vi "Main.vi"(8 "error in (no error)":errorcluster, 11 "ModuleAdmin":refnum<class "ModuleAdmin.lvclass">) -> ()   [LabVIEW 2018, in "FgenModule.lvlib"]
uses:
  FgenModule.lvlib
  <userlib>/NIST/ModuleAdminLib/ModuleAdmin/ModuleAdmin.lvclass
  C:/Program Files (x86)/National Instruments/LabVIEW 2018/user.lib/NIST/ModuleAdminLib/ModuleAdminBase/ModuleAdminBase.lvclass
  PublicAPI/Arguments/Requests/clStopArgument.ctl
  FgenPlugins/FgenPluginBaseClass/FgenPluginsBase.lvclass
  C:/Program Files (x86)/National Instruments/LabVIEW 2018/user.lib/NIST/BaseClasses/BasePlugin_class/BasePlugin.lvclass
  <userlib>/NIST/ModuleAdminLib/ModuleAdmin/ModuleAdmin.lvclass/ModuleAdmin.ctl
  FgenPlugins/FgenPluginBaseClass/FgenPluginsBase.lvclass/FgenPluginsBase.ctl
  MemberClasses/FunctionBaseClass/FunctionBase.lvclass/FunctionBase.ctl
  FgenPlugins/TypeDefs/clTriggers.ctl
  FgenPlugins/TypeDefs/Trigger.ctl
  FgenPlugins/TypeDefs/TriggerType.ctl
  <userlib>/NIST/BaseClasses/BasePlugin_class/BasePlugin.lvclass/BasePlugin.ctl
  FgenPlugins/TypeDefs/InitOptions.ctl
  FgenPlugins/TypeDefs/Channels.ctl
  FgenPlugins/TypeDefs/Channel.ctl
  <vilib>/Utility/error.llb/DialogType.ctl
  <userlib>/NIST/ModuleAdminLib/ModuleAdmin/Accessors/Read ShowPanel_.vi
  <userlib>/NIST/ModuleAdminLib/ModuleAdmin/Accessors/Write ShowPanel_.vi
  FgenPlugins/FgenPluginBaseClass/Accessors/Read FunctionClass.vi
  FgenPlugins/FgenPluginBaseClass/Accessors/Write FunctionClass.vi
  MemberClasses/FunctionBaseClass/Accessors/Write Waveforms.vi
  MemberClasses/FunctionBaseClass/Accessors/Read Waveforms.vi
  FgenPlugins/FgenPluginBaseClass/Accessors/Write Triggers.vi
  FgenPlugins/FgenPluginBaseClass/Read Triggers.vi
  <userlib>/NIST/BaseClasses/BasePlugin_class/Accessors/Read PluginIniFilePath.vi
  <userlib>/NIST/ModuleAdminLib/ModuleAdmin/Accessors/Read CloneRegRef.vi
  <extravilib>/ChannelInstances/Tag-bool/Read With Abort.vi
  <extravilib>/ChannelInstances/Tag-bool/Write With Abort.vi
  <extravilib>/ChannelInstances/Tag-bool/Instantiate.vi
  <extravilib>/ChannelInstances/Tag-bool/EndpointRead.vi
  <vilib>/Utility/error.llb/Error Cluster From Error Code.vi
  <extravilib>/ChannelInstances/Tag-bool/Endpoint.vi
  <vilib>/ErrorRing/Error Ring.xnode
  MemberClasses/FunctionBaseClass/FunctionBase.lvclass
  <userlib>/NIST/ModuleAdminLib/CloneRegistration/CloneRegistration.lvclass
  <userlib>/NIST/BaseClasses/Object_class/BaseObject.lvclass
  <userlib>/NIST/ModuleAdminLib/ModuleAdmin.lvlib
  FgenPlugins/FgenPlugins.lvlib
  <extravilib>/ChannelInstances/Tag-bool.lvlib
panel:
  out "error out":errorcluster
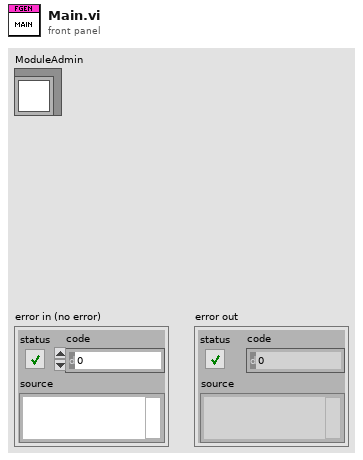
[diagram p1: front panel]
types:
  T1 = typedef "FgenModule.lvlib/clRequestEvents.ctl" = cluster{"StopRequest":refnum<user-event>, "PathToINI":refnum<user-event>, " LoadPlugin":refnum<user-event>, "ShowPanel":refnum<user-event>, "Initialize":refnum<user-event>, "GetChannels":refnum<user-event>, "SetChannels":refnum<user-event>, "Abort":refnum<user-event>, "Initiate":refnum<user-event>, "ConfigDlg":refnum<user-event>, "GetFunction":refnum<user-event>, "SetFunction":refnum<user-event>, "ConfigFunction":refnum<user-event>, "GetWfrm":refnum<user-event>, "SetWfrm":refnum<user-event>, "GetTriggers":refnum<user-event>, "SetTriggers":refnum<user-event>, "ConfigTriggers":refnum<user-event>, "Close":refnum<user-event>, "GetFunctionParams":refnum<user-event>, "SetFunctionParams":refnum<user-event>, "GetFunctionArbs":refnum<user-event>, "SetFunctionArbs":refnum<user-event>, "GetFunctionSampleRate":refnum<user-event>, "SetFunctionSampleRate":refnum<user-event>}
  T2 = typedef "FgenModule.lvlib/clBroadcastEvents.ctl" = cluster{"DidInit":refnum<user-event>, "StatusUpdate":refnum<user-event>, "ErrorReport":refnum<user-event>, "DidStop":refnum<user-event>, "PathToINI":refnum<user-event>, "Channels":refnum<user-event>, "Function":refnum<user-event>, "Waveforms":refnum<user-event>, "Triggers":refnum<user-event>, "FunctionParams":refnum<user-event>, "FunctionArbs":refnum<user-event>, "FunctionSampleRate":refnum<user-event>}
  T3 = typedef "FgenModule.lvlib/clStopArgument.ctl" = cluster{"Exit via Stop Module Req?":bool, "Wait for Module to stop?":bool, "ModuleAdmin":refnum<class "ModuleAdmin.lvclass">}
  T4 = enum32{"Invalid", "Standard", "Closed", "Hidden", "Minimized", "Maximized"}
  T5 = typedef "FgenPlugins.lvlib/clTriggers.ctl" = cluster{"Count":i32, "Triggers":T6[]}
  T6 = typedef "FgenPlugins.lvlib/Trigger.ctl" = cluster{"Source":string, "Slope":enum16{"Positive", "Negative", "Either"}, "Threshold":dbl, "Delay":dbl, "TriggerType":T7}
  T7 = typedef "FgenPlugins.lvlib/TriggerType.ctl" = enum16{"None", "Start", "Stop", "Hold", "Resume", "Advance"}
  T8 = typedef "FgenPlugins.lvlib/InitOptions.ctl" = cluster{"IDQuery":bool, "Reset":bool}
  T9 = typedef "FgenPlugins.lvlib/Channels.ctl" = cluster{"Count":u16, "Channel":T10[]}
  T10 = typedef "FgenPlugins.lvlib/Channel.ctl" = cluster{"Name":string, "Enabled":bool, "Operation":enum16{"Continuous", "Burst"}, "Impedance (50)":dbl, "Handle":string, "Connected":bool, "Mode (Function)":enum16{"Function", "Arbitrary", "Sequence"}}
  T11 = typedef "Tag-bool.lvlib/))Channel.ctl" = refnum<queue>
  T12 = typedef "DialogType.ctl" = u16
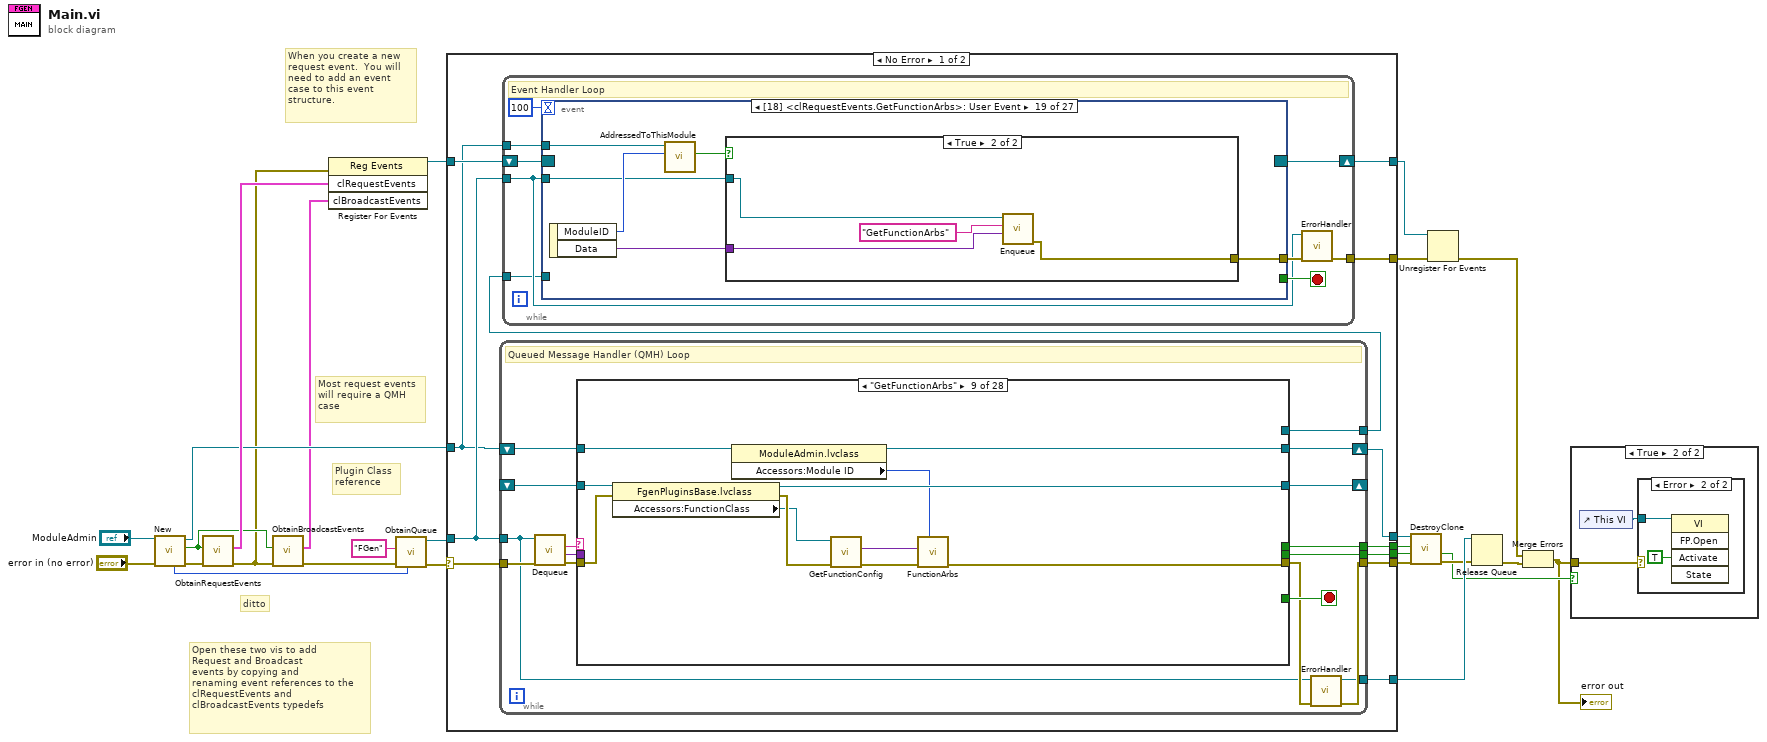
[diagram p0: block diagram]
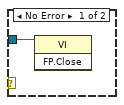
[diagram p3: hidden frame]
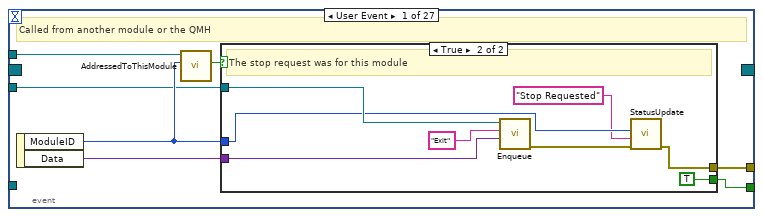
[diagram p4: hidden frame]
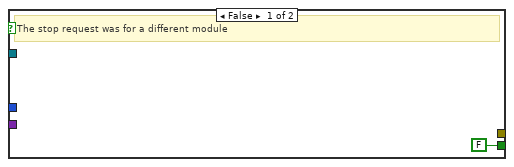
[diagram p5: hidden frame]
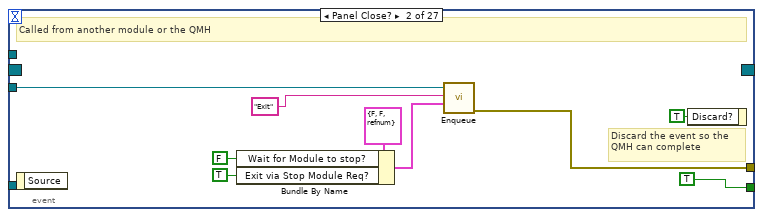
[diagram p6: hidden frame]
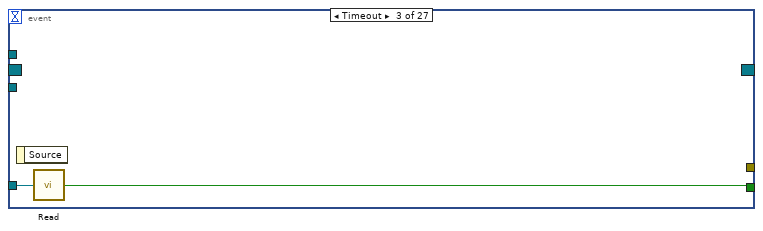
[diagram p7: hidden frame]
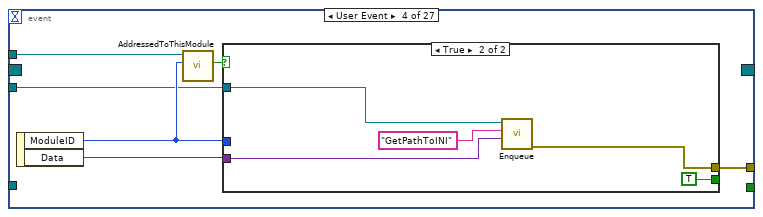
[diagram p8: hidden frame]
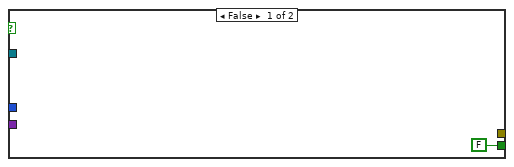
[diagram p9: hidden frame]
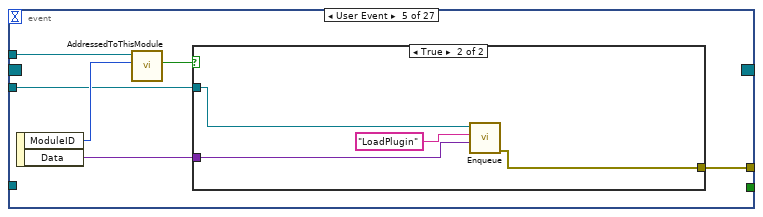
[diagram p10: hidden frame]
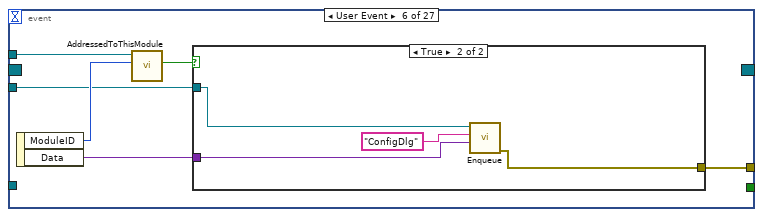
[diagram p12: hidden frame]
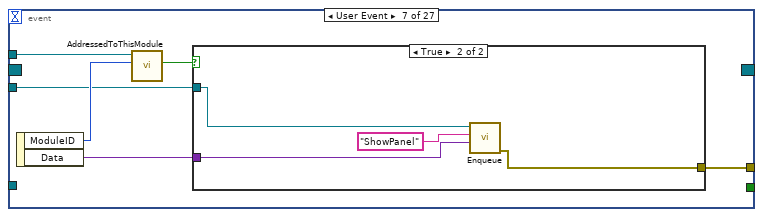
[diagram p14: hidden frame]
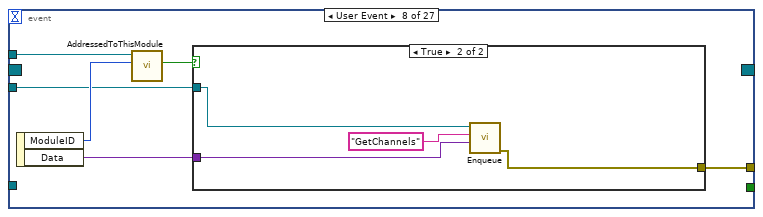
[diagram p16: hidden frame]
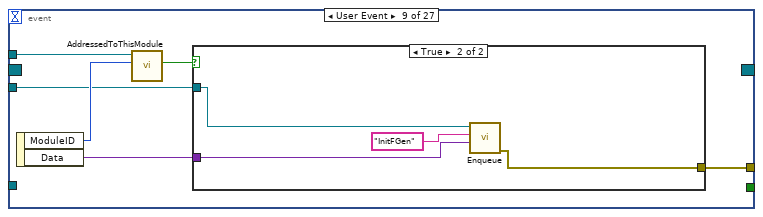
[diagram p18: hidden frame]
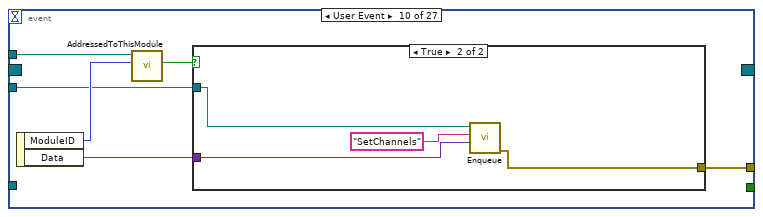
[diagram p20: hidden frame]
diagram:
  # "Plugin Class\nreference"
  # "Open these two vis to add\nRequest and Broadcast \nevents by copying and \nrenaming event references to the \nclRequestEvents and \nclBroadcastEvents typedefs"
  # "ditto"
  # "Most request events\nwill require a QMH\ncase"
  # "When you create a new request event.  You will need to add an event case to this event structure."
  n1 = call <userlib>:"New.vi"("error in (no error)"="error in (no error)", "ModuleAdmin"="ModuleAdmin") -> ("error out"=w24:errorcluster, "First?"=w17:bool, "ModuleAdmin"=w20:refnum<class "ModuleAdmin.lvclass">, "Module ID"=w6:i32)  [unwired: 6 in]
  n2 = call "ObtainRequestEvents.vi"("error in (no error)"=w24, "CreateNew (F)"=w17) -> ("error out"=w16:errorcluster, "clRequestEvents"=w23:T1)  [unwired: 8 in]
  n3 = call "ObtainBroadcastEvents.vi"("error in (no error)"=w16, "CreateNew? (F)"=w17) -> ("error out"=w18:errorcluster, "clBroadcastEvents"=w15:T2)  [unwired: 8 in]
  n4 = register-events(error in=w16, w23, w15) -> (reference out=w14:refnum<event-registration>)  [unwired: 1 in, 1 out]
  n5 = call "ObtainQueue.vi"("Module ID"=w6, "error in (no error)"=w18, "ModuleName"="FGen") -> ("error out"=w22:errorcluster, "MessageQueue"=w21:refnum<queue>)  [unwired: 7 in]
  n6 = case shown="No Error" w22 {
    selector: w22 -> [w38 w759]
    tunnel: w21 -> [w36 w756]
    tunnel: w20 -> [w33 w757]
    tunnel: [w37 w751] -> w13
    tunnel: [w35 w756] -> w19
    tunnel: w14 -> [w34 w752]
    tunnel: [w32 w755] -> w11
    tunnel: [w31 _] -> w10
    tunnel: [w30 _] -> w9
    tunnel: [w29 w751] -> w4
    tunnel: [w27 w752] -> w3
    frame No Error {
      n7 = while {
        tunnel: w36 -> [w318]
        tunnel: w38 -> [w331]
        tunnel: [w324] -> w37
        tunnel: [w317] -> w35
        tunnel: [w326] -> w31
        tunnel: [w325] -> w30
        shift-right: [w322] -> _
        shift-left: _ -> [w321]
        shift-right: [w320] -> w32
        shift-left: w33 -> [w327]
        tunnel: [w319] -> w28
        stop <- w332 stop-if-true
        # "Queued Message Handler (QMH) Loop"
        n8 = call "Dequeue.vi"("error in (no error)"=w331, "MessageQueue"=w318) -> ("error out"=w330:errorcluster, "Message Data"=w328:variant, "Message"=w329:string)  [unwired: 6 in, 1 out]
        n9 = case shown="\"GetFunctionArbs\"" w329 {
          selector: w329 -> [_ _ _ _ _ _ _ _ _ _ _ _ _ _ _ _ _ _ _ _ _ _ _ _ _ _ _ w739]
          tunnel: [_ _ _ _ _ _ _ _ _ _ _ _ _ _ _ _ _ _ _ _ _ _ _ _ _ w717 _ _] -> w332
          tunnel: w327 -> [w353 w370 w381 w428 w442 w449 w479 w497 w508 w519 w534 w549 w564 w582 w593 w605 w615 w622 w631 w648 w663 w670 w678 w687 w698 w711 w720 w742]
          tunnel: [w342 w363 w382 w422 w440 w445 w470 w492 w499 w513 w531 w546 w561 w571 w591 w596 w609 w617 w632 w641 w654 w664 w675 w684 w699 w716 w721 w738] -> w323
          tunnel: w330 -> [_ w373 w390 w427 w436 w455 w477 w495 w506 w517 w525 w540 w555 w578 w589 w604 w611 w623 w627 w650 w660 w672 w680 w689 w693 w707 w729 _]
          tunnel: w328 -> [_ w372 w392 _ _ w450 _ _ _ _ w527 w542 w557 w577 _ w603 _ _ _ w649 w661 _ _ _ _ w715 w728 _]
          tunnel: [_ _ _ _ _ _ _ _ _ _ _ _ _ _ _ _ _ _ _ _ _ _ _ _ _ w713 _ _] -> w326
          tunnel: [_ _ _ _ _ _ _ _ _ _ _ _ _ _ _ _ _ _ _ _ _ _ _ _ _ w712 _ _] -> w325
          tunnel: [refnum<class "FgenPluginsBase.lvclass"> refnum ("MyPlugins.lvlib:MyPluginsBase.lvclass") w362 w380 w425 w435 w444 w469 w491 w504 w515 w521 w536 w551 w570 w585 w594 w607 w621 w628 w634 w658 w667 w679 w688 w696 w710 w719 w736] -> w322
          tunnel: w321 -> [_ w362 w377 w426 w437 w457 w478 w496 w507 w518 w529 w544 w559 w580 w590 w606 w613 w624 w630 w647 w659 w671 w681 w690 w697 w709 w719 w736]
          tunnel: [w333 w369 w378 w424 w441 w443 w474 w494 w505 w516 w533 w548 w563 w581 w583 w595 w608 w620 w625 w640 w653 w666 w677 w686 w695 w705 w718 w735] -> w320
          tunnel: [_ _ _ _ _ _ _ _ _ _ _ _ _ _ _ _ _ _ _ _ _ _ _ _ _ w700 _ _] -> w319
          frame "Initialize" {
            # "Initialize is always called after ObtainQueue.vi is run"
            n10 = property class="ModuleAdmin.lvclass"(reference=w353) -> (reference out=w339:refnum<class "ModuleAdmin.lvclass">, error out=w350:errorcluster, "Accessors:Module ID"=w341:i32, "Accessors:ShowPanel_"=w336:bool, "Accessors:External Launch"=w335:bool, "Accessors:ModuleName"=w337:string)  [unwired: 1 in]
            n11 = Compound Arithmetic op=OR(w336, invert w335) -> (w334:bool)
            n12 = Select(t=T4."Standard" ("Front Panel Window:State"), s=w334, f=T4."Hidden" ("Front Panel Window:State")) -> (s? t:f=w346:T4)
            n13 = invoke class="VI" method="FP.Open"(error in=w350, "State"=w346) -> (error out=w349:errorcluster)  [unwired: 3 in, 4 out]
            n14 = call <userlib>:"ModuleName.vi"("Name"=w337, "ModuleID"=w341) -> ("ModuleName"=w345:string)  [unwired: 9 in]
            n15 = property class="VI"(error in=w349, "Front Panel.Title"=w345) -> (reference out=w352:refnum<vi>, error out=w351:errorcluster)  [unwired: 1 in]
            n16 = invoke class="VI" method="FP.Center"(reference=w352, error in=w351) -> (error out=w340:errorcluster)  [unwired: 1 in, 2 out]
            n17 = case shown="True" w335 {
              tunnel: [w354 w360] -> w343
              tunnel: [w355 w357] -> w333
              tunnel: w340 -> [w354 w359]
              tunnel: w339 -> [w355 w356]
              frame False {
              }
              frame True {
                n18 = call <userlib>:"WaitOnModuleSync.vi"("error in (no error)"=w359, "ModuleAdmin"=w356) -> ("error out"=w361:errorcluster, "ModuleAdmin"=w358:refnum<class "ModuleAdmin.lvclass">)  [unwired: 8 in]
                n19 = call <userlib>:"WaitOnEventSync.vi"("error in (no error)"=w361, "ModuleAdmin"=w358) -> ("error out"=w360:errorcluster, "ModuleAdmin"=w357:refnum<class "ModuleAdmin.lvclass">)  [unwired: 8 in]
              }
            }
            n20 = call "DidInit.vi"("Init?"=TRUE, "error in (no error)"=w343, "ModuleAdmin"=w333) -> ("error out"=w342:errorcluster)  [unwired: 8 in]
          }
          frame "ShowPanel" {
            n21 = Variant To Data(error in=w373, type=TRUE, Variant=w372) -> (data=w365:bool, error out=w368:errorcluster)
            n22 = Select(t=T4."Standard" ("Front Panel Window:State"), s=w365, f=T4."Hidden" ("Front Panel Window:State")) -> (s? t:f=w364:T4)
            n23 = property class="VI"(error in=w368, "FP.State"=w364) -> (error out=w363:errorcluster)  [unwired: 1 in, 1 out]
            n24 = property class="ModuleAdmin.lvclass"(reference=w370, "Accessors:ShowPanel_"=w365) -> (reference out=w369:refnum<class "ModuleAdmin.lvclass">)  [unwired: 1 in, 1 out]
          }
          frame "LoadPlugin" {
            n25 = Variant To Data(error in=w390, type=path "", Variant=w392) -> (data=w379:path, error out=w375:errorcluster)
            n26 = call-dynamic "Close.vi"("error in (no error)"=w375, "FgenPluginsBase in"=w377) -> ("error out"=w374:errorcluster, "FgenPluginsBase out"=w376:refnum<class "FgenPluginsBase.lvclass">)  [unwired: 8 in]
            n27 = call <userlib>:"GetPathToClass.vi"("error in (no error)"=w374, "configuration file path"=w379) -> ("error IO"=w386:errorcluster, "PathToClass"=w389:path)  [unwired: 8 in]
            n28 = Current VI's Path() -> (path=w388:path)
            n29 = Build Path(base path=w388, name or relative path=w389) -> (appended path=w387:path)
            n30 = call <vilib>:"Check if File or Folder Exists.vi"("error in (no error)"=w386, "path"=w387) -> ("error out"=w383:errorcluster, "file or folder exists?"=w385:bool, "dup path"=w384:path)  [unwired: 7 in]
            n31 = case shown="True" w385 {
              tunnel: w384 -> [w396 w411]
              tunnel: w383 -> [_ w419]
              tunnel: [w395 w414] -> w382
              tunnel: w381 -> [w393 w413]
              tunnel: w376 -> [w394 _]
              tunnel: [w394 w406] -> w380
              tunnel: w379 -> [_ w407]
              tunnel: [w393 w410] -> w378
              frame False {
                n32 = Path To String(path=w396) -> (string=w397:string)
                n33 = xnode "Error Ring"("parameter 0"=w397) -> ("error out"=w395:errorcluster)
              }
              frame True {
                n34 = call-dynamic "LoadClassFromFile.vi"("error in (no error)"=w419, "class path"=w411, "reference in"=refnum<class "FgenPluginsBase.lvclass"> refnum ("MyPlugins.lvlib:MyPluginsBase.lvclass")) -> ("error out"=w409:errorcluster, "reference out"=w408:refnum<class "FgenPluginsBase.lvclass">)  [unwired: 7 in]
                n35 = property class="ModuleAdmin.lvclass"(reference=w413) -> (reference out=w410:refnum<class "ModuleAdmin.lvclass">, "Accessors:Module ID"=w412:i32)  [unwired: 1 in, 1 out]
                n36 = call-dynamic "GetDefaultParams.vi"("error in (no error)"=w409, "Path"=w407, "FgenPluginsBase in"=w408) -> ("error out"=w405:errorcluster, "FgenPluginsBase out"=w406:refnum<class "FgenPluginsBase.lvclass">)  [unwired: 7 in]
                n37 = Path To String(path=w411) -> (string=w416:string)
                n38 = Format Into String(format string="Plugin %s loaded ", w416) -> (resulting string=w415:string)  [unwired: 2 in, 1 out]
                n39 = call "StatusUpdate.vi"("error in (no error)"=w405, "Status"=w415, "ModuleID"=w412) -> ("error out"=w414:errorcluster)  [unwired: 8 in]
              }
            }
          }
          frame "ConfigDlg" {
            n40 = call-dynamic "ConfigDlg.vi"("error in (no error)"=w427, "FgenPluginsBase in"=w426) -> ("error out"=w423:errorcluster, "Changed"=w420:bool, "FgenPluginsBase out"=w425:refnum<class "FgenPluginsBase.lvclass">)  [unwired: 7 in]
            n41 = property class="ModuleAdmin.lvclass"(reference=w428) -> (reference out=w424:refnum<class "ModuleAdmin.lvclass">, "Accessors:Module ID"=w421:i32)  [unwired: 1 in, 1 out]
            n42 = case shown="True" w420 {
              tunnel: w423 -> [w429 w433]
              tunnel: [w429 w432] -> w422
              tunnel: w421 -> [_ w431]
              frame False {
              }
              frame True {
                n43 = call "StatusUpdate.vi"("error in (no error)"=w433, "Status"="Configuration Updated", "ModuleID"=w431) -> ("error out"=w432:errorcluster)  [unwired: 8 in]
              }
            }
          }
          frame "ConfigFunction" {
            n44 = call-dynamic "ConfigFunction.vi"("error in (no error)"=w436, "FgenPluginsBase in"=w437) -> ("error out"=w434:errorcluster, "FgenPluginsBase out"=w435:refnum<class "FgenPluginsBase.lvclass">)  [unwired: 8 in]
            n45 = property class="ModuleAdmin.lvclass"(reference=w442) -> (reference out=w441:refnum<class "ModuleAdmin.lvclass">, "Accessors:Module ID"=w439:i32)  [unwired: 1 in, 1 out]
            n46 = call "StatusUpdate.vi"("error in (no error)"=w434, "Status"="Function Configured", "ModuleID"=w439) -> ("error out"=w440:errorcluster)  [unwired: 8 in]
          }
          frame "SetFunction" {
            n47 = property class="FgenPluginsBase.lvclass"(reference=w457, error in=w455) -> (reference out=w456:refnum<class "FgenPluginsBase.lvclass">, error out=w453:errorcluster, "Accessors:FunctionClass"=w454:refnum<class "FunctionBase.lvclass">)
            n48 = disable-structure shown="Enabled" {
              disable-tunnel: w454 -> [w462 w466]
              disable-tunnel: w453 -> [w461 w465]
              disable-tunnel: [w460 w464] -> w452
              disable-tunnel: [w459 w463] -> w451
              disable-tunnel: w450 -> [w458 w467]
              frame Disabled {
                n49 = call-dynamic "SetConfig.vi"("error in (no error)"=w461, "Variant"=w458, "FunctionBase in"=w462) -> ("error out"=w460:errorcluster, "FunctionBase out"=w459:refnum<class "FunctionBase.lvclass">)  [unwired: 7 in]
              }
              frame Enabled {
                n50 = Variant To Data(error in=w465, type=w466, Variant=w467) -> (data=w463:refnum<class "FunctionBase.lvclass">, error out=w464:errorcluster)
              }
            }
            n51 = property class="FgenPluginsBase.lvclass"(reference=w456, error in=w452, "Accessors:FunctionClass"=w451) -> (reference out=w444:refnum<class "FgenPluginsBase.lvclass">, error out=w446:errorcluster)
            n52 = property class="ModuleAdmin.lvclass"(reference=w449) -> (reference out=w443:refnum<class "ModuleAdmin.lvclass">, "Accessors:Module ID"=w447:i32)  [unwired: 1 in, 1 out]
            n53 = call "StatusUpdate.vi"("error in (no error)"=w446, "Status"="Function Set", "ModuleID"=w447) -> ("error out"=w445:errorcluster)  [unwired: 8 in]
          }
          frame "GetFunction" {
            n54 = property class="FgenPluginsBase.lvclass"(reference=w478, error in=w477) -> (reference out=w469:refnum<class "FgenPluginsBase.lvclass">, error out=w475:errorcluster, "Accessors:FunctionClass"=w476:refnum<class "FunctionBase.lvclass">)
            n55 = property class="ModuleAdmin.lvclass"(reference=w479) -> (reference out=w474:refnum<class "ModuleAdmin.lvclass">, "Accessors:Module ID"=w473:i32)  [unwired: 1 in, 1 out]
            n56 = disable-structure shown="Enabled" {
              disable-tunnel: w476 -> [w483 w485]
              disable-tunnel: w475 -> [w482 w484]
              disable-tunnel: [w481 w485] -> w472
              disable-tunnel: [w480 w484] -> w471
              frame Disabled {
                n57 = call-dynamic "GetConfig.vi"("error in (no error)"=w482, "FunctionBase in"=w483) -> ("error out"=w480:errorcluster, "Config"=w481:variant)  [unwired: 7 in, 1 out]
              }
              frame Enabled {
              }
            }
            n58 = To Variant(anything=w472) -> (Variant=w468:variant)
            n59 = call "Function.vi"("ModuleID"=w473, "error in (no error)"=w471, "Function"=w468) -> ("error out"=w470:errorcluster)  [unwired: 8 in]
          }
          frame "GetFunctionParams" {
            n60 = property class="FgenPluginsBase.lvclass"(reference=w496, error in=w495) -> (reference out=w491:refnum<class "FgenPluginsBase.lvclass">, error out=w488:errorcluster, "Accessors:FunctionClass"=w487:refnum<class "FunctionBase.lvclass">)
            n61 = property class="ModuleAdmin.lvclass"(reference=w497) -> (reference out=w494:refnum<class "ModuleAdmin.lvclass">, "Accessors:Module ID"=w493:i32)  [unwired: 1 in, 1 out]
            n62 = call-dynamic "GetSignalParams.vi"("error in (no error)"=w488, "FunctionBase in"=w487) -> ("error out"=w489:errorcluster, "Params"=w486:variant)  [unwired: 7 in, 1 out]
            n63 = To Variant(anything=w486) -> (Variant=w490:variant)
            n64 = call "FunctionParams.vi"("ModuleID"=w493, "error in (no error)"=w489, "Function"=w490) -> ("error out"=w492:errorcluster)  [unwired: 8 in]
          }
          frame "GetFunctionArbs" {
            n65 = property class="FgenPluginsBase.lvclass"(reference=w507, error in=w506) -> (reference out=w504:refnum<class "FgenPluginsBase.lvclass">, error out=w503:errorcluster, "Accessors:FunctionClass"=w502:refnum<class "FunctionBase.lvclass">)
            n66 = property class="ModuleAdmin.lvclass"(reference=w508) -> (reference out=w505:refnum<class "ModuleAdmin.lvclass">, "Accessors:Module ID"=w501:i32)  [unwired: 1 in, 1 out]
            n67 = call-dynamic "GetFunctionConfig.vi"("error in (no error)"=w503, "FunctionBase In"=w502) -> ("error out"=w500:errorcluster, "FunctionConfig"=w498:variant)  [unwired: 7 in, 1 out]
            n68 = call "FunctionArbs.vi"("ModuleID"=w501, "error in (no error)"=w500, "Function"=w498) -> ("error out"=w499:errorcluster)  [unwired: 8 in]
          }
          frame "GetFunctionSampleRate" {
            n69 = property class="FgenPluginsBase.lvclass"(reference=w518, error in=w517) -> (reference out=w515:refnum<class "FgenPluginsBase.lvclass">, error out=w512:errorcluster, "Accessors:FunctionClass"=w511:refnum<class "FunctionBase.lvclass">)
            n70 = property class="ModuleAdmin.lvclass"(reference=w519) -> (reference out=w516:refnum<class "ModuleAdmin.lvclass">, "Accessors:Module ID"=w514:i32)  [unwired: 1 in, 1 out]
            n71 = call-dynamic "GetFunctionSampleRate.vi"("error in (no error)"=w512, "FunctionBase in"=w511) -> ("error out"=w509:errorcluster, "SampleRate"=w510:variant)  [unwired: 7 in, 1 out]
            n72 = call "FunctionSampleRate.vi"("ModuleID"=w514, "error in (no error)"=w509, "SampleRate"=w510) -> ("error out"=w513:errorcluster)  [unwired: 8 in]
          }
          frame "SetFunctionParams" {
            n73 = property class="FgenPluginsBase.lvclass"(reference=w529, error in=w525) -> (reference out=w526:refnum<class "FgenPluginsBase.lvclass">, error out=w524:errorcluster, "Accessors:FunctionClass"=w528:refnum<class "FunctionBase.lvclass">)
            n74 = call-dynamic "SetSignalParams.vi"("error in (no error)"=w524, "Variant"=w527, "FunctionBase in"=w528) -> ("error out"=w522:errorcluster, "FunctionBase out"=w523:refnum<class "FunctionBase.lvclass">)  [unwired: 7 in]
            n75 = property class="FgenPluginsBase.lvclass"(reference=w526, error in=w522, "Accessors:FunctionClass"=w523) -> (reference out=w521:refnum<class "FgenPluginsBase.lvclass">, error out=w520:errorcluster)
            n76 = property class="ModuleAdmin.lvclass"(reference=w534) -> (reference out=w533:refnum<class "ModuleAdmin.lvclass">, "Accessors:Module ID"=w532:i32)  [unwired: 1 in, 1 out]
            n77 = call "StatusUpdate.vi"("error in (no error)"=w520, "Status"="Set FunctionParams", "ModuleID"=w532) -> ("error out"=w531:errorcluster)  [unwired: 8 in]
          }
          frame "SetFunctionArbs" {
            n78 = property class="FgenPluginsBase.lvclass"(reference=w544, error in=w540) -> (reference out=w541:refnum<class "FgenPluginsBase.lvclass">, error out=w539:errorcluster, "Accessors:FunctionClass"=w543:refnum<class "FunctionBase.lvclass">)
            n79 = call-dynamic "SetFunctionArbs.vi"("error in (no error)"=w539, "Variant"=w542, "FunctionBase in"=w543) -> ("error out"=w537:errorcluster, "FunctionBase out"=w538:refnum<class "FunctionBase.lvclass">)  [unwired: 7 in]
            n80 = property class="FgenPluginsBase.lvclass"(reference=w541, error in=w537, "Accessors:FunctionClass"=w538) -> (reference out=w536:refnum<class "FgenPluginsBase.lvclass">, error out=w535:errorcluster)
            n81 = property class="ModuleAdmin.lvclass"(reference=w549) -> (reference out=w548:refnum<class "ModuleAdmin.lvclass">, "Accessors:Module ID"=w547:i32)  [unwired: 1 in, 1 out]
            n82 = call "StatusUpdate.vi"("error in (no error)"=w535, "Status"="Set FunctionArbs", "ModuleID"=w547) -> ("error out"=w546:errorcluster)  [unwired: 8 in]
          }
          frame "SetFunctionSampleRate" {
            n83 = property class="FgenPluginsBase.lvclass"(reference=w559, error in=w555) -> (reference out=w556:refnum<class "FgenPluginsBase.lvclass">, error out=w554:errorcluster, "Accessors:FunctionClass"=w558:refnum<class "FunctionBase.lvclass">)
            n84 = call-dynamic "SetFunctionSampleRate.vi"("error in (no error)"=w554, "SampleRate"=w557, "FunctionBase in"=w558) -> ("error out"=w552:errorcluster, "FunctionBase out"=w553:refnum<class "FunctionBase.lvclass">)  [unwired: 7 in]
            n85 = property class="FgenPluginsBase.lvclass"(reference=w556, error in=w552, "Accessors:FunctionClass"=w553) -> (reference out=w551:refnum<class "FgenPluginsBase.lvclass">, error out=w550:errorcluster)
            n86 = property class="ModuleAdmin.lvclass"(reference=w564) -> (reference out=w563:refnum<class "ModuleAdmin.lvclass">, "Accessors:Module ID"=w562:i32)  [unwired: 1 in, 1 out]
            n87 = call "StatusUpdate.vi"("error in (no error)"=w550, "Status"="Set FunctionSampleRate", "ModuleID"=w562) -> ("error out"=w561:errorcluster)  [unwired: 8 in]
          }
          frame "SetWfrm" {
            n88 = Variant To Data(error in=w578, type=waveform(dbl)[] [] ("Waveforms"), Variant=w577) -> (data=w575:waveform(dbl)[], error out=w574:errorcluster)
            n89 = property class="FgenPluginsBase.lvclass"(reference=w580, error in=w574) -> (reference out=w566:refnum<class "FgenPluginsBase.lvclass">, error out=w573:errorcluster, "Accessors:FunctionClass"=w579:refnum<class "FunctionBase.lvclass">)
            n90 = property class="FunctionBase.lvclass"(reference=w579, error in=w573, "Accessors:Waveforms"=w575) -> (reference out=w569:refnum<class "FunctionBase.lvclass">, error out=w567:errorcluster)
            n91 = property class="FgenPluginsBase.lvclass"(reference=w566, error in=w567, "Accessors:FunctionClass"=w569) -> (reference out=w570:refnum<class "FgenPluginsBase.lvclass">, error out=w565:errorcluster)
            n92 = property class="ModuleAdmin.lvclass"(reference=w582) -> (reference out=w581:refnum<class "ModuleAdmin.lvclass">, "Accessors:Module ID"=w568:i32)  [unwired: 1 in, 1 out]
            n93 = call "StatusUpdate.vi"("error in (no error)"=w565, "Status"="Waveforms Set", "ModuleID"=w568) -> ("error out"=w571:errorcluster)  [unwired: 8 in]
          }
          frame "GetWfrm" {
            n94 = property class="FgenPluginsBase.lvclass"(reference=w590, error in=w589) -> (reference out=w585:refnum<class "FgenPluginsBase.lvclass">, error out=w584:errorcluster, "Accessors:FunctionClass"=w588:refnum<class "FunctionBase.lvclass">)
            n95 = property class="FunctionBase.lvclass"(reference=w588, error in=w584) -> (error out=w586:errorcluster, "Accessors:Waveforms"=w587:waveform(dbl)[])  [unwired: 1 out]
            n96 = property class="ModuleAdmin.lvclass"(reference=w593) -> (reference out=w583:refnum<class "ModuleAdmin.lvclass">, "Accessors:Module ID"=w592:i32)  [unwired: 1 in, 1 out]
            n97 = call "Waveforms.vi"("ModuleID"=w592, "error in (no error)"=w586, "Waveforms"=w587) -> ("error out"=w591:errorcluster)  [unwired: 8 in]
          }
          frame "SetTriggers" {
            n98 = Variant To Data(error in=w604, type=T5 {"Count"=0, "Triggers"=[]} ("Triggers"), Variant=w603) -> (data=w601:T5, error out=w600:errorcluster)
            n99 = property class="FgenPluginsBase.lvclass"(reference=w606, error in=w600, "Accessors:Triggers"=w601) -> (reference out=w594:refnum<class "FgenPluginsBase.lvclass">, error out=w597:errorcluster)
            n100 = property class="ModuleAdmin.lvclass"(reference=w605) -> (reference out=w595:refnum<class "ModuleAdmin.lvclass">, "Accessors:Module ID"=w598:i32)  [unwired: 1 in, 1 out]
            n101 = call "StatusUpdate.vi"("error in (no error)"=w597, "Status"="Triggers Updated", "ModuleID"=w598) -> ("error out"=w596:errorcluster)  [unwired: 8 in]
          }
          frame "GetTriggers" {
            n102 = property class="ModuleAdmin.lvclass"(reference=w615) -> (reference out=w608:refnum<class "ModuleAdmin.lvclass">, "Accessors:Module ID"=w614:i32)  [unwired: 1 in, 1 out]
            n103 = property class="FgenPluginsBase.lvclass"(reference=w613, error in=w611) -> (reference out=w607:refnum<class "FgenPluginsBase.lvclass">, error out=w610:errorcluster, "Accessors:Triggers"=w612:T5)
            n104 = call "Triggers.vi"("ModuleID"=w614, "error in (no error)"=w610, "Triggers"=w612) -> ("error out"=w609:errorcluster)  [unwired: 8 in]
          }
          frame "ConfigTriggers" {
            n105 = property class="ModuleAdmin.lvclass"(reference=w622) -> (reference out=w620:refnum<class "ModuleAdmin.lvclass">, "Accessors:Module ID"=w616:i32)  [unwired: 1 in, 1 out]
            n106 = call-dynamic "ConfigTriggers.vi"("error in (no error)"=w623, "FgenPluginsBase in"=w624) -> ("error out"=w618:errorcluster, "FgenPluginsBase out"=w621:refnum<class "FgenPluginsBase.lvclass">)  [unwired: 8 in]
            n107 = call "StatusUpdate.vi"("error in (no error)"=w618, "Status"="Triggers Configured", "ModuleID"=w616) -> ("error out"=w617:errorcluster)  [unwired: 8 in]
          }
          frame "GetPathToINI" {
            n108 = property class="FgenPluginsBase.lvclass"(reference=w630, error in=w627) -> (reference out=w628:refnum<class "FgenPluginsBase.lvclass">, error out=w626:errorcluster, "Accessors:PluginIniFilePath"=w629:path)
            n109 = property class="ModuleAdmin.lvclass"(reference=w631) -> (reference out=w625:refnum<class "ModuleAdmin.lvclass">, "Accessors:Module ID"=w633:i32)  [unwired: 1 in, 1 out]
            n110 = call "PathToINIBroadcast.vi"("error in (no error)"=w626, "PathToINI"=w629, "ModuleID"=w633) -> ("error out"=w632:errorcluster)  [unwired: 8 in]
          }
          frame "InitFGen" {
            n111 = Variant To Data(error in=w650, type=T8 {"IDQuery"=FALSE, "Reset"=FALSE} ("InitOptions"), Variant=w649) -> (data=w645:T8, error out=w642:errorcluster)
            n112 = Unbundle By Name(w645) -> ("IDQuery"=w644:bool, "Reset"=w643:bool)
            n113 = call-dynamic "Initialize.vi"("error in (no error)"=w642, "Reset (F)"=w643, "IdQuery (F)"=w644, "FgenPluginsBase in"=w647) -> ("error out"=w637:errorcluster, "FgenPluginsBase out"=w636:refnum<class "FgenPluginsBase.lvclass">)  [unwired: 6 in]
            n114 = call-dynamic "ConfigClock.vi"("error in (no error)"=w637, "FgenPluginsBase in"=w636) -> ("error out"=w635:errorcluster, "FgenPluginsBase out"=w634:refnum<class "FgenPluginsBase.lvclass">)  [unwired: 8 in]
            n115 = property class="ModuleAdmin.lvclass"(reference=w648) -> (reference out=w640:refnum<class "ModuleAdmin.lvclass">, "Accessors:Module ID"=w639:i32)  [unwired: 1 in, 1 out]
            n116 = call "StatusUpdate.vi"("error in (no error)"=w635, "Status"="Device Initialized", "ModuleID"=w639) -> ("error out"=w641:errorcluster)  [unwired: 8 in]
          }
          frame "SetChannels" {
            n117 = Variant To Data(error in=w660, type=T9 {"Count"=0, "Channel"=[]} ("Channels"), Variant=w661) -> (data=w656:T9, error out=w657:errorcluster)
            n118 = call-dynamic "SetChannels.vi"("error in (no error)"=w657, "Channels"=w656, "FgenPluginsBase in"=w659) -> ("error out"=w655:errorcluster, "FgenPluginsBase out"=w658:refnum<class "FgenPluginsBase.lvclass">)  [unwired: 7 in]
            n119 = property class="ModuleAdmin.lvclass"(reference=w663) -> (reference out=w653:refnum<class "ModuleAdmin.lvclass">, "Accessors:Module ID"=w652:i32)  [unwired: 1 in, 1 out]
            n120 = call "StatusUpdate.vi"("error in (no error)"=w655, "Status"="Channels Updated", "ModuleID"=w652) -> ("error out"=w654:errorcluster)  [unwired: 8 in]
          }
          frame "InitGen" {
            n121 = call-dynamic "InitiateGeneration.vi"("error in (no error)"=w672, "FgenPluginsBase in"=w671) -> ("error out"=w669:errorcluster, "FgenPluginsBase out"=w667:refnum<class "FgenPluginsBase.lvclass">)  [unwired: 8 in]
            n122 = property class="ModuleAdmin.lvclass"(reference=w670) -> (reference out=w666:refnum<class "ModuleAdmin.lvclass">, "Accessors:Module ID"=w668:i32)  [unwired: 1 in, 1 out]
            n123 = call "StatusUpdate.vi"("error in (no error)"=w669, "Status"="Initiate Generation", "ModuleID"=w668) -> ("error out"=w664:errorcluster)  [unwired: 8 in]
          }
          frame "AbortGen" {
            n124 = call-dynamic "AbortGeneration.vi"("error in (no error)"=w680, "FgenPluginsBase in"=w681) -> ("error out"=w676:errorcluster, "FgenPluginsBase out"=w679:refnum<class "FgenPluginsBase.lvclass">)  [unwired: 8 in]
            n125 = property class="ModuleAdmin.lvclass"(reference=w678) -> (reference out=w677:refnum<class "ModuleAdmin.lvclass">, "Accessors:Module ID"=w674:i32)  [unwired: 1 in, 1 out]
            n126 = call "StatusUpdate.vi"("error in (no error)"=w676, "Status"="Abort Generation", "ModuleID"=w674) -> ("error out"=w675:errorcluster)  [unwired: 8 in]
          }
          frame "Close" {
            n127 = call-dynamic "Close.vi"("error in (no error)"=w689, "FgenPluginsBase in"=w690) -> ("error out"=w685:errorcluster, "FgenPluginsBase out"=w688:refnum<class "FgenPluginsBase.lvclass">)  [unwired: 8 in]
            n128 = property class="ModuleAdmin.lvclass"(reference=w687) -> (reference out=w686:refnum<class "ModuleAdmin.lvclass">, "Accessors:Module ID"=w683:i32)  [unwired: 1 in, 1 out]
            n129 = call "StatusUpdate.vi"("error in (no error)"=w685, "Status"="Closed", "ModuleID"=w683) -> ("error out"=w684:errorcluster)  [unwired: 8 in]
          }
          frame "GetChannels" {
            n130 = property class="ModuleAdmin.lvclass"(reference=w698) -> (reference out=w695:refnum<class "ModuleAdmin.lvclass">, "Accessors:Module ID"=w694:i32)  [unwired: 1 in, 1 out]
            n131 = call-dynamic "GetChannels.vi"("error in (no error)"=w693, "FgenPluginsBase in"=w697) -> ("error out"=w692:errorcluster, "Channels"=w691:cluster{"Count":u16, "Channel":T10[]}, "FgenPluginsBase out"=w696:refnum<class "FgenPluginsBase.lvclass">)  [unwired: 7 in]
            n132 = call "Channels.vi"("ModuleID"=w694, "error in (no error)"=w692, "Channels"=w691) -> ("error out"=w699:errorcluster)  [unwired: 8 in]
          }
          frame "Exit" {
            w717 = TRUE
            # "Called by the StopRequest event handler case"
            n133 = property class="ModuleAdmin.lvclass"(reference=w711) -> (reference out=w705:refnum<class "ModuleAdmin.lvclass">, "Accessors:Module ID"=w704:i32)  [unwired: 1 in, 1 out]
            n134 = call-dynamic "AbortGeneration.vi"("error in (no error)"=w707, "FgenPluginsBase in"=w709) -> ("error out"=w706:errorcluster, "FgenPluginsBase out"=w708:refnum<class "FgenPluginsBase.lvclass">)  [unwired: 8 in]
            n135 = call-dynamic "Close.vi"("error in (no error)"=w706, "FgenPluginsBase in"=w708) -> ("error out"=w702:errorcluster, "FgenPluginsBase out"=w710:refnum<class "FgenPluginsBase.lvclass">)  [unwired: 8 in]
            n136 = call "StatusUpdate.vi"("error in (no error)"=w702, "Status"="Exiting", "ModuleID"=w704) -> ("error out"=w701:errorcluster)  [unwired: 8 in]
            n137 = control-ref of="This VI"() -> (w714:refnum<vi>)
            n138 = call "HandleExit.vi"("error in (no error)"=w701, "VI Refnum"=w714, "StopArgument"=w715, "ModuleAdmin"=w705) -> ("error out"=w716:errorcluster, "Exit via Stop Module Req?"=w712:bool, "WaitForStop?"=w713:bool)  [unwired: 5 in]
            n139 = call <extravilib>:"Write.vi"("element"=w717) -> ("channel"=w700:T11)  [unwired: 1 out]
          }
          frame "Error" {
            n140 = property class="ModuleAdmin.lvclass"(reference=w720) -> (reference out=w718:refnum<class "ModuleAdmin.lvclass">, "Accessors:External Launch"=w724:bool, "Accessors:Module ID"=w722:i32)  [unwired: 1 in, 1 out]
            n141 = Variant To Data(error in=w729, type=errorcluster {"status"=FALSE, "code"=0, "source"=""} ("error constant"), Variant=w728) -> (data=w723:errorcluster, error out=w726:errorcluster)
            n142 = call "ReportError.vi"("error in (no error)"=w726, "ErrorReported"=w723, "ModuleID"=w722) -> ("error out"=w725:errorcluster)  [unwired: 8 in]
            n143 = case shown="True" w724 {
              tunnel: w725 -> [w733 w734]
              tunnel: w723 -> [w732 _]
              tunnel: [w731 w734] -> w721
              tunnel: w720 -> [w730 _]
              frame False {
                # "Todo:  Add an event to ask the user\nIf the module should stop or continue"
                # "Stand alone: now, force an exit"
                n144 = call <vilib>:"Simple Error Handler.vi"("error in (no error)"=w732) -> ()  [unwired: 4 in, 5 out]
                n145 = call "StopRequest.vi"("error in (no error)"=w733, "ModuleAdmin"=w730) -> ("error out"=w731:errorcluster)  [unwired: 8 in, 1 out]
              }
              frame True {
                # "Externally launched modules only broadcast the error msg"
              }
            }
          }
          frame Default {
            # "Called only if a message was queued and no QMH case was created"
            n146 = property class="ModuleAdmin.lvclass"(reference=w742) -> (reference out=w735:refnum<class "ModuleAdmin.lvclass">, "Accessors:Module ID"=w741:i32, "Accessors:ModuleName"=w737:string)  [unwired: 1 in, 1 out]
            n147 = call <userlib>:"ModuleName.vi"("Name"=w737, "ModuleID"=w741) -> ("ModuleName"=w740:string)  [unwired: 9 in]
            n148 = xnode "Error Ring"("parameter 0"=w739, "parameter 1"=w740) -> ("error out"=w738:errorcluster)
          }
        }
        n149 = call "ErrorHandler.vi"("error in (no error)"=w323, "MessageQueue"=w318) -> ("error out"=w324:errorcluster, "MessageQueue"=w317:refnum<queue>)  [unwired: 8 in]
      }
      n150 = while {
        tunnel: w36 -> [w41]
        shift-right: [w45] -> w27
        shift-left: w34 -> [w46]
        tunnel: w33 -> [w44]
        tunnel: [w42] -> w29
        tunnel: w28 -> [w39]
        stop <- w47 stop-if-true
        # "Event Handler Loop"
        n151 = event shown="[18] <clRequestEvents.GetFunctionArbs>: User Event" {
          selector: w46 -> [_ _ _ _ _ _ _ _ _ _ _ _ _ _ _ _ _ _ _ _ _ _ _ _ _ _ _]
          dyn-events: [_ _ _ _ _ _ _ _ _ _ _ _ _ _ _ _ _ _ _ _ _ _ _ _ _ _ _] -> w45
          timeout: 100 -> [_ _ _ _ _ _ _ _ _ _ _ _ _ _ _ _ _ _ _ _ _ _ _ _ _ _ _]
          tunnel: w41 -> [w51 w72 _ w77 w88 w98 w108 w118 w128 w138 w148 w158 w168 w178 w188 w198 w208 w218 w228 w238 w248 w258 w268 w278 w288 w298 w308]
          tunnel: [w50 TRUE w73 _ _ _ _ _ _ _ _ _ _ _ _ _ _ _ _ _ _ _ _ _ _ _ _] -> w47
          tunnel: w44 -> [w54 _ _ w76 w92 w102 w112 w122 w132 w142 w152 w162 w172 w182 w192 w202 w212 w222 w232 w242 w252 w262 w272 w282 w292 w302 w312]
          tunnel: [w49 w70 _ w75 w89 w99 w109 w119 w129 w139 w149 w159 w169 w179 w189 w199 w209 w219 w229 w239 w249 w259 w269 w279 w289 w299 w309] -> w43
          tunnel: w39 -> [_ _ w74 _ _ _ _ _ _ _ _ _ _ _ _ _ _ _ _ _ _ _ _ _ _ _ _]
          event User Event {
            # "Called from another module or the QMH"
            n152 = event-data() -> ("ModuleID"=w52:i32, "Data"=w48:variant)  [unwired: 1 in]
            n153 = call <userlib>:"AddressedToThisModule.vi"("ModuleID"=w52, "ModuleAdmin"=w54) -> ("AddressedToThisInstance?"=w53:bool)  [unwired: 8 in, 1 out]
            n154 = case shown="True" w53 {
              tunnel: w52 -> [_ w57]
              tunnel: w51 -> [_ w63]
              tunnel: [FALSE TRUE] -> w50
              tunnel: [_ w58] -> w49
              tunnel: w48 -> [_ w60]
              frame False {
                # "The stop request was for a different module"
              }
              frame True {
                # "The stop request was for this module"
                n155 = call "Enqueue.vi"("Message Data"=w60, "Message"="Exit", "MessageQueue"=w63) -> ("error out"=w59:errorcluster)  [unwired: 7 in, 1 out]
                n156 = call "StatusUpdate.vi"("error in (no error)"=w59, "Status"="Stop Requested", "ModuleID"=w57) -> ("error out"=w58:errorcluster)  [unwired: 8 in]
              }
            }
          }
          event Panel Close? {
            # "Discard the event so the QMH can complete"
            # "Called from another module or the QMH"
            n157 = event-data() -> ()  [unwired: 1 in, 1 out]
            n158 = Bundle By Name(cluster=T3 {"Exit via Stop Module Req?"=FALSE, "Wait for Module to stop?"=FALSE, "ModuleAdmin"=refnum} ("Stop Argument"), "Wait for Module to stop?"=FALSE, "Exit via Stop Module Req?"=TRUE) -> (w67:T3)
            n159 = call "Enqueue.vi"("Message Data"=w67, "Message"="Exit", "MessageQueue"=w72) -> ("error out"=w70:errorcluster)  [unwired: 7 in, 1 out]
            n160 = event-data("Discard?"=TRUE) -> ()  [unwired: 1 in, 1 out]
          }
          event Timeout {
            n161 = event-data() -> ()  [unwired: 1 in, 1 out]
            n162 = call <extravilib>:"Read.vi"("channel"=w74) -> ("element"=w73:bool)  [unwired: 1 in, 1 out]
          }
          event User Event {
            n163 = event-data() -> ("ModuleID"=w78:i32, "Data"=w79:variant)  [unwired: 1 in]
            n164 = call <userlib>:"AddressedToThisModule.vi"("ModuleID"=w78, "ModuleAdmin"=w76) -> ("AddressedToThisInstance?"=w80:bool)  [unwired: 8 in, 1 out]
            n165 = case shown="True" w80 {
              tunnel: w78 -> [_ _]
              tunnel: w77 -> [_ w86]
              tunnel: [FALSE TRUE] -> _
              tunnel: [_ w84] -> w75
              tunnel: w79 -> [_ w82]
              frame False {
                # "The stop request was for a different module"
              }
              frame True {
                # "The stop request was for this module"
                n166 = call "Enqueue.vi"("Message Data"=w82, "Message"="GetPathToINI", "MessageQueue"=w86) -> ("error out"=w84:errorcluster)  [unwired: 7 in, 1 out]
              }
            }
          }
          event User Event {
            n167 = event-data() -> ("ModuleID"=w91:i32, "Data"=w87:variant)  [unwired: 1 in]
            n168 = call <userlib>:"AddressedToThisModule.vi"("ModuleID"=w91, "ModuleAdmin"=w92) -> ("AddressedToThisInstance?"=w90:bool)  [unwired: 8 in, 1 out]
            n169 = case shown="True" w90 {
              tunnel: [_ w93] -> w89
              tunnel: w88 -> [_ w96]
              tunnel: w87 -> [_ w94]
              frame False {
              }
              frame True {
                n170 = call "Enqueue.vi"("Message Data"=w94, "Message"="LoadPlugin", "MessageQueue"=w96) -> ("error out"=w93:errorcluster)  [unwired: 7 in, 1 out]
              }
            }
          }
          event User Event {
            n171 = event-data() -> ("ModuleID"=w101:i32, "Data"=w97:variant)  [unwired: 1 in]
            n172 = call <userlib>:"AddressedToThisModule.vi"("ModuleID"=w101, "ModuleAdmin"=w102) -> ("AddressedToThisInstance?"=w100:bool)  [unwired: 8 in, 1 out]
            n173 = case shown="True" w100 {
              tunnel: [_ w103] -> w99
              tunnel: w98 -> [_ w106]
              tunnel: w97 -> [_ w104]
              frame False {
              }
              frame True {
                n174 = call "Enqueue.vi"("Message Data"=w104, "Message"="ConfigDlg", "MessageQueue"=w106) -> ("error out"=w103:errorcluster)  [unwired: 7 in, 1 out]
              }
            }
          }
          event User Event {
            n175 = event-data() -> ("ModuleID"=w111:i32, "Data"=w107:variant)  [unwired: 1 in]
            n176 = call <userlib>:"AddressedToThisModule.vi"("ModuleID"=w111, "ModuleAdmin"=w112) -> ("AddressedToThisInstance?"=w110:bool)  [unwired: 8 in, 1 out]
            n177 = case shown="True" w110 {
              tunnel: [_ w113] -> w109
              tunnel: w108 -> [_ w116]
              tunnel: w107 -> [_ w114]
              frame False {
              }
              frame True {
                n178 = call "Enqueue.vi"("Message Data"=w114, "Message"="ShowPanel", "MessageQueue"=w116) -> ("error out"=w113:errorcluster)  [unwired: 7 in, 1 out]
              }
            }
          }
          event User Event {
            n179 = event-data() -> ("ModuleID"=w121:i32, "Data"=w117:variant)  [unwired: 1 in]
            n180 = call <userlib>:"AddressedToThisModule.vi"("ModuleID"=w121, "ModuleAdmin"=w122) -> ("AddressedToThisInstance?"=w120:bool)  [unwired: 8 in, 1 out]
            n181 = case shown="True" w120 {
              tunnel: [_ w123] -> w119
              tunnel: w118 -> [_ w126]
              tunnel: w117 -> [_ w124]
              frame False {
              }
              frame True {
                n182 = call "Enqueue.vi"("Message Data"=w124, "Message"="GetChannels", "MessageQueue"=w126) -> ("error out"=w123:errorcluster)  [unwired: 7 in, 1 out]
              }
            }
          }
          event User Event {
            n183 = event-data() -> ("ModuleID"=w131:i32, "Data"=w127:variant)  [unwired: 1 in]
            n184 = call <userlib>:"AddressedToThisModule.vi"("ModuleID"=w131, "ModuleAdmin"=w132) -> ("AddressedToThisInstance?"=w130:bool)  [unwired: 8 in, 1 out]
            n185 = case shown="True" w130 {
              tunnel: [_ w133] -> w129
              tunnel: w128 -> [_ w136]
              tunnel: w127 -> [_ w134]
              frame False {
              }
              frame True {
                n186 = call "Enqueue.vi"("Message Data"=w134, "Message"="InitFGen", "MessageQueue"=w136) -> ("error out"=w133:errorcluster)  [unwired: 7 in, 1 out]
              }
            }
          }
          event User Event {
            n187 = event-data() -> ("ModuleID"=w141:i32, "Data"=w137:variant)  [unwired: 1 in]
            n188 = call <userlib>:"AddressedToThisModule.vi"("ModuleID"=w141, "ModuleAdmin"=w142) -> ("AddressedToThisInstance?"=w140:bool)  [unwired: 8 in, 1 out]
            n189 = case shown="True" w140 {
              tunnel: [_ w143] -> w139
              tunnel: w138 -> [_ w146]
              tunnel: w137 -> [_ w144]
              frame False {
              }
              frame True {
                n190 = call "Enqueue.vi"("Message Data"=w144, "Message"="SetChannels", "MessageQueue"=w146) -> ("error out"=w143:errorcluster)  [unwired: 7 in, 1 out]
              }
            }
          }
          event User Event {
            n191 = event-data() -> ("ModuleID"=w151:i32, "Data"=w147:variant)  [unwired: 1 in]
            n192 = call <userlib>:"AddressedToThisModule.vi"("ModuleID"=w151, "ModuleAdmin"=w152) -> ("AddressedToThisInstance?"=w150:bool)  [unwired: 8 in, 1 out]
            n193 = case shown="True" w150 {
              tunnel: [_ w153] -> w149
              tunnel: w148 -> [_ w156]
              tunnel: w147 -> [_ w154]
              frame False {
              }
              frame True {
                n194 = call "Enqueue.vi"("Message Data"=w154, "Message"="InitGen", "MessageQueue"=w156) -> ("error out"=w153:errorcluster)  [unwired: 7 in, 1 out]
              }
            }
          }
          event User Event {
            n195 = event-data() -> ("ModuleID"=w161:i32, "Data"=w157:variant)  [unwired: 1 in]
            n196 = call <userlib>:"AddressedToThisModule.vi"("ModuleID"=w161, "ModuleAdmin"=w162) -> ("AddressedToThisInstance?"=w160:bool)  [unwired: 8 in, 1 out]
            n197 = case shown="True" w160 {
              tunnel: [_ w163] -> w159
              tunnel: w158 -> [_ w166]
              tunnel: w157 -> [_ w164]
              frame False {
              }
              frame True {
                n198 = call "Enqueue.vi"("Message Data"=w164, "Message"="AbortGen", "MessageQueue"=w166) -> ("error out"=w163:errorcluster)  [unwired: 7 in, 1 out]
              }
            }
          }
          event User Event {
            n199 = event-data() -> ("ModuleID"=w171:i32, "Data"=w167:variant)  [unwired: 1 in]
            n200 = call <userlib>:"AddressedToThisModule.vi"("ModuleID"=w171, "ModuleAdmin"=w172) -> ("AddressedToThisInstance?"=w170:bool)  [unwired: 8 in, 1 out]
            n201 = case shown="True" w170 {
              tunnel: [_ w173] -> w169
              tunnel: w168 -> [_ w176]
              tunnel: w167 -> [_ w174]
              frame False {
              }
              frame True {
                n202 = call "Enqueue.vi"("Message Data"=w174, "Message"="ConfigFunction", "MessageQueue"=w176) -> ("error out"=w173:errorcluster)  [unwired: 7 in, 1 out]
              }
            }
          }
          event User Event {
            n203 = event-data() -> ("ModuleID"=w181:i32, "Data"=w177:variant)  [unwired: 1 in]
            n204 = call <userlib>:"AddressedToThisModule.vi"("ModuleID"=w181, "ModuleAdmin"=w182) -> ("AddressedToThisInstance?"=w180:bool)  [unwired: 8 in, 1 out]
            n205 = case shown="True" w180 {
              tunnel: [_ w183] -> w179
              tunnel: w178 -> [_ w186]
              tunnel: w177 -> [_ w184]
              frame False {
              }
              frame True {
                n206 = call "Enqueue.vi"("Message Data"=w184, "Message"="SetFunction", "MessageQueue"=w186) -> ("error out"=w183:errorcluster)  [unwired: 7 in, 1 out]
              }
            }
          }
          event User Event {
            n207 = event-data() -> ("ModuleID"=w191:i32, "Data"=w187:variant)  [unwired: 1 in]
            n208 = call <userlib>:"AddressedToThisModule.vi"("ModuleID"=w191, "ModuleAdmin"=w192) -> ("AddressedToThisInstance?"=w190:bool)  [unwired: 8 in, 1 out]
            n209 = case shown="True" w190 {
              tunnel: [_ w193] -> w189
              tunnel: w188 -> [_ w196]
              tunnel: w187 -> [_ w194]
              frame False {
              }
              frame True {
                n210 = call "Enqueue.vi"("Message Data"=w194, "Message"="GetFunction", "MessageQueue"=w196) -> ("error out"=w193:errorcluster)  [unwired: 7 in, 1 out]
              }
            }
          }
          event User Event {
            n211 = event-data() -> ("ModuleID"=w201:i32, "Data"=w197:variant)  [unwired: 1 in]
            n212 = call <userlib>:"AddressedToThisModule.vi"("ModuleID"=w201, "ModuleAdmin"=w202) -> ("AddressedToThisInstance?"=w200:bool)  [unwired: 8 in, 1 out]
            n213 = case shown="True" w200 {
              tunnel: [_ w203] -> w199
              tunnel: w198 -> [_ w206]
              tunnel: w197 -> [_ w204]
              frame False {
              }
              frame True {
                n214 = call "Enqueue.vi"("Message Data"=w204, "Message"="GetFunctionParams", "MessageQueue"=w206) -> ("error out"=w203:errorcluster)  [unwired: 7 in, 1 out]
              }
            }
          }
          event User Event {
            n215 = event-data() -> ("ModuleID"=w211:i32, "Data"=w207:variant)  [unwired: 1 in]
            n216 = call <userlib>:"AddressedToThisModule.vi"("ModuleID"=w211, "ModuleAdmin"=w212) -> ("AddressedToThisInstance?"=w210:bool)  [unwired: 8 in, 1 out]
            n217 = case shown="True" w210 {
              tunnel: [_ w213] -> w209
              tunnel: w208 -> [_ w216]
              tunnel: w207 -> [_ w214]
              frame False {
              }
              frame True {
                n218 = call "Enqueue.vi"("Message Data"=w214, "Message"="SetFunctionParams", "MessageQueue"=w216) -> ("error out"=w213:errorcluster)  [unwired: 7 in, 1 out]
              }
            }
          }
          event User Event {
            n219 = event-data() -> ("ModuleID"=w221:i32, "Data"=w217:variant)  [unwired: 1 in]
            n220 = call <userlib>:"AddressedToThisModule.vi"("ModuleID"=w221, "ModuleAdmin"=w222) -> ("AddressedToThisInstance?"=w220:bool)  [unwired: 8 in, 1 out]
            n221 = case shown="True" w220 {
              tunnel: [_ w223] -> w219
              tunnel: w218 -> [_ w226]
              tunnel: w217 -> [_ w224]
              frame False {
              }
              frame True {
                n222 = call "Enqueue.vi"("Message Data"=w224, "Message"="SetFunctionArbs", "MessageQueue"=w226) -> ("error out"=w223:errorcluster)  [unwired: 7 in, 1 out]
              }
            }
          }
          event User Event {
            n223 = event-data() -> ("ModuleID"=w231:i32, "Data"=w227:variant)  [unwired: 1 in]
            n224 = call <userlib>:"AddressedToThisModule.vi"("ModuleID"=w231, "ModuleAdmin"=w232) -> ("AddressedToThisInstance?"=w230:bool)  [unwired: 8 in, 1 out]
            n225 = case shown="True" w230 {
              tunnel: [_ w233] -> w229
              tunnel: w228 -> [_ w236]
              tunnel: w227 -> [_ w234]
              frame False {
              }
              frame True {
                n226 = call "Enqueue.vi"("Message Data"=w234, "Message"="GetFunctionArbs", "MessageQueue"=w236) -> ("error out"=w233:errorcluster)  [unwired: 7 in, 1 out]
              }
            }
          }
          event User Event {
            n227 = event-data() -> ("ModuleID"=w241:i32, "Data"=w237:variant)  [unwired: 1 in]
            n228 = call <userlib>:"AddressedToThisModule.vi"("ModuleID"=w241, "ModuleAdmin"=w242) -> ("AddressedToThisInstance?"=w240:bool)  [unwired: 8 in, 1 out]
            n229 = case shown="True" w240 {
              tunnel: [_ w243] -> w239
              tunnel: w238 -> [_ w246]
              tunnel: w237 -> [_ w244]
              frame False {
              }
              frame True {
                n230 = call "Enqueue.vi"("Message Data"=w244, "Message"="GetFunctionSampleRate", "MessageQueue"=w246) -> ("error out"=w243:errorcluster)  [unwired: 7 in, 1 out]
              }
            }
          }
          event User Event {
            n231 = event-data() -> ("ModuleID"=w251:i32, "Data"=w247:variant)  [unwired: 1 in]
            n232 = call <userlib>:"AddressedToThisModule.vi"("ModuleID"=w251, "ModuleAdmin"=w252) -> ("AddressedToThisInstance?"=w250:bool)  [unwired: 8 in, 1 out]
            n233 = case shown="True" w250 {
              tunnel: [_ w253] -> w249
              tunnel: w248 -> [_ w256]
              tunnel: w247 -> [_ w254]
              frame False {
              }
              frame True {
                n234 = call "Enqueue.vi"("Message Data"=w254, "Message"="SetFunctionSampleRate", "MessageQueue"=w256) -> ("error out"=w253:errorcluster)  [unwired: 7 in, 1 out]
              }
            }
          }
          event User Event {
            n235 = event-data() -> ("ModuleID"=w261:i32, "Data"=w257:variant)  [unwired: 1 in]
            n236 = call <userlib>:"AddressedToThisModule.vi"("ModuleID"=w261, "ModuleAdmin"=w262) -> ("AddressedToThisInstance?"=w260:bool)  [unwired: 8 in, 1 out]
            n237 = case shown="True" w260 {
              tunnel: [_ w263] -> w259
              tunnel: w258 -> [_ w266]
              tunnel: w257 -> [_ w264]
              frame False {
              }
              frame True {
                n238 = call "Enqueue.vi"("Message Data"=w264, "Message"="SetWfrm", "MessageQueue"=w266) -> ("error out"=w263:errorcluster)  [unwired: 7 in, 1 out]
              }
            }
          }
          event User Event {
            n239 = event-data() -> ("ModuleID"=w271:i32, "Data"=w267:variant)  [unwired: 1 in]
            n240 = call <userlib>:"AddressedToThisModule.vi"("ModuleID"=w271, "ModuleAdmin"=w272) -> ("AddressedToThisInstance?"=w270:bool)  [unwired: 8 in, 1 out]
            n241 = case shown="True" w270 {
              tunnel: [_ w273] -> w269
              tunnel: w268 -> [_ w276]
              tunnel: w267 -> [_ w274]
              frame False {
              }
              frame True {
                n242 = call "Enqueue.vi"("Message Data"=w274, "Message"="GetWfrm", "MessageQueue"=w276) -> ("error out"=w273:errorcluster)  [unwired: 7 in, 1 out]
              }
            }
          }
          event User Event {
            n243 = event-data() -> ("ModuleID"=w281:i32, "Data"=w277:variant)  [unwired: 1 in]
            n244 = call <userlib>:"AddressedToThisModule.vi"("ModuleID"=w281, "ModuleAdmin"=w282) -> ("AddressedToThisInstance?"=w280:bool)  [unwired: 8 in, 1 out]
            n245 = case shown="True" w280 {
              tunnel: [_ w283] -> w279
              tunnel: w278 -> [_ w286]
              tunnel: w277 -> [_ w284]
              frame False {
              }
              frame True {
                n246 = call "Enqueue.vi"("Message Data"=w284, "Message"="SetTriggers", "MessageQueue"=w286) -> ("error out"=w283:errorcluster)  [unwired: 7 in, 1 out]
              }
            }
          }
          event User Event {
            n247 = event-data() -> ("ModuleID"=w291:i32, "Data"=w287:variant)  [unwired: 1 in]
            n248 = call <userlib>:"AddressedToThisModule.vi"("ModuleID"=w291, "ModuleAdmin"=w292) -> ("AddressedToThisInstance?"=w290:bool)  [unwired: 8 in, 1 out]
            n249 = case shown="True" w290 {
              tunnel: [_ w293] -> w289
              tunnel: w288 -> [_ w296]
              tunnel: w287 -> [_ w294]
              frame False {
              }
              frame True {
                n250 = call "Enqueue.vi"("Message Data"=w294, "Message"="GetTriggers", "MessageQueue"=w296) -> ("error out"=w293:errorcluster)  [unwired: 7 in, 1 out]
              }
            }
          }
          event User Event {
            n251 = event-data() -> ("ModuleID"=w301:i32, "Data"=w297:variant)  [unwired: 1 in]
            n252 = call <userlib>:"AddressedToThisModule.vi"("ModuleID"=w301, "ModuleAdmin"=w302) -> ("AddressedToThisInstance?"=w300:bool)  [unwired: 8 in, 1 out]
            n253 = case shown="True" w300 {
              tunnel: [_ w303] -> w299
              tunnel: w298 -> [_ w306]
              tunnel: w297 -> [_ w304]
              frame False {
              }
              frame True {
                n254 = call "Enqueue.vi"("Message Data"=w304, "Message"="ConfigTriggers", "MessageQueue"=w306) -> ("error out"=w303:errorcluster)  [unwired: 7 in, 1 out]
              }
            }
          }
          event User Event {
            n255 = event-data() -> ("ModuleID"=w311:i32, "Data"=w307:variant)  [unwired: 1 in]
            n256 = call <userlib>:"AddressedToThisModule.vi"("ModuleID"=w311, "ModuleAdmin"=w312) -> ("AddressedToThisInstance?"=w310:bool)  [unwired: 8 in, 1 out]
            n257 = case shown="True" w310 {
              tunnel: [_ w313] -> w309
              tunnel: w308 -> [_ w316]
              tunnel: w307 -> [_ w314]
              frame False {
              }
              frame True {
                n258 = call "Enqueue.vi"("Message Data"=w314, "Message"="Close", "MessageQueue"=w316) -> ("error out"=w313:errorcluster)  [unwired: 7 in, 1 out]
              }
            }
          }
        }
        n259 = call "ErrorHandler.vi"("error in (no error)"=w43, "MessageQueue"=w41) -> ("error out"=w42:errorcluster)  [unwired: 8 in, 1 out]
      }
    }
    frame Error {
      n260 = property class="ModuleAdmin.lvclass"(reference=w757) -> (reference out=w755:refnum<class "ModuleAdmin.lvclass">, "Accessors:CloneRegRef"=w754:refnum<data-value>, "Accessors:Module ID"=w753:i32)  [unwired: 1 in, 1 out]
      n261 = call <userlib>:"Remove.vi"("Module ID"=w753, "CloneRegRef"=w754) -> ("error out"=w758:errorcluster)  [unwired: 7 in, 2 out]
      n262 = flat-sequence {
        tunnel: w759 -> [w762]
        tunnel: w758 -> [_]
        tunnel: [w760] -> w751
        frame #0 {
          w761 = T12 2 items=["no dialog", "OK message", "continue or stop message", "OK message + warnings", "continue/stop + warnings"] ("type of dialog (OK msg:1)")
          n263 = call <vilib>:"Simple Error Handler.vi"("type of dialog (OK msg:1)"=w761, "error in (no error)"=w762) -> ("error out"=w760:errorcluster)  [unwired: 3 in, 4 out]
        }
      }
    }
  }
  n264 = call "DestroyClone.vi"("error in (no error)"=w13, "Exit via Stop Module Req?"=w9, "Wait for Module to stop?"=w10, "ModuleAdmin"=w11) -> ("error out"=w12:errorcluster, "External Launch"=w8:bool)  [unwired: 5 in, 1 out]
  n265 = Unregister For Events(event registration refnum=w3, error in=w4) -> (error out=w1:errorcluster)
  n266 = Release Queue(queue=w19, error in (no error)=w12) -> (error out=w7:errorcluster)  [unwired: 1 in, 2 out]
  n267 = Merge Errors(w1, w7) -> (w2:errorcluster)
  "error out" <- w2
  n268 = case shown="True" w8 {
    tunnel: w2 -> [_ w764]
    frame False {
    }
    frame True {
      n269 = control-ref of="This VI"() -> (w763:refnum<vi>)
      n270 = case shown="Error" w764 {
        tunnel: w763 -> [w765 w766]
        frame No Error {
          n271 = invoke class="VI" method="FP.Close"(reference=w765) -> ()  [unwired: 2 in, 3 out]
        }
        frame Error {
          n272 = invoke class="VI" method="FP.Open"(reference=w766, "Activate"=TRUE ("Activate?")) -> ()  [unwired: 3 in, 5 out]
        }
      }
    }
  }
